vi "FTW-CodeGen-Image.vi"(0 "State In":T1, 5 "XRef":refnum<vi>) -> (4 "Image":picture)   [LabVIEW 2012, in "FTW-JSON-Serialize.xnode"]
uses:
  FTW-JSON-Serialize.xnode
  FTW-CodeGen-State.ctl
panel:
  # "Inputs"
  # "Outputs"
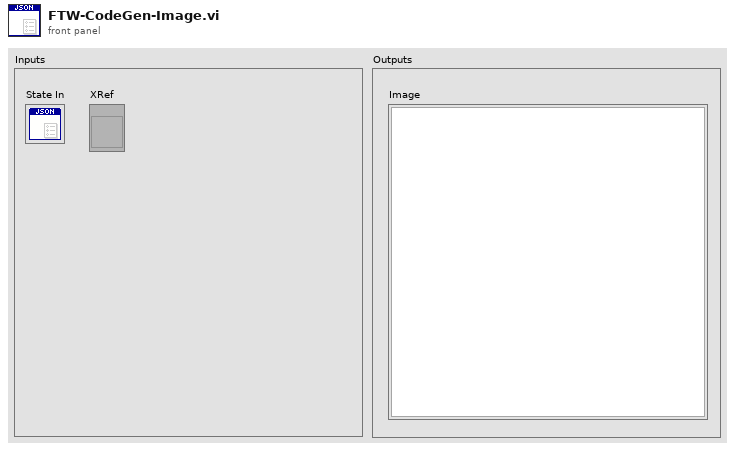
[diagram p1: front panel]
types:
  T1 = typedef "FTW-JSON-Serialize.xnode/FTW-CodeGen-State.ctl" = cluster{"Prototype Filepath":path}
  T2 = typedef "imagedata.ctl" = cluster{"image type":i32, "image depth":i32, "image":u8[], "mask":u8[], "colors":u32[], "Rectangle":cluster{"left":i16, "top":i16, "right":i16, "bottom":i16}}
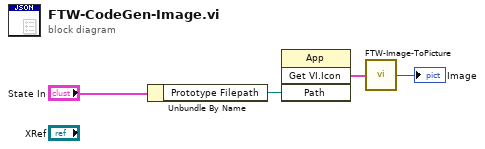
[diagram p0: block diagram]
diagram:
  n1 = Unbundle By Name("State In") -> ("Prototype Filepath"=w2:path)
  n2 = invoke class="App" method="Get VI.Icon"("Path"=w2) -> ("Get VI.Icon"=w1:T2)  [unwired: 3 in, 3 out]
  n3 = call "FTW-Image-ToPicture.vi"("Image"=w1) -> ("Picture"=→"Image":picture)
